vi "rest_get_latest.vi"(8 "error in (no error)":errorcluster, 11 "Base URL":string="http://localhost:5001/") -> (0 "error out":errorcluster, 2 "value":T1)   [LabVIEW 2024]
uses:
  <vilib>/addons/_JKI.lib/REST Client/classes/REST Client/REST Client.lvclass
  TypeDefs/MeasurementData.ctl
panel:
  out "Response body":string
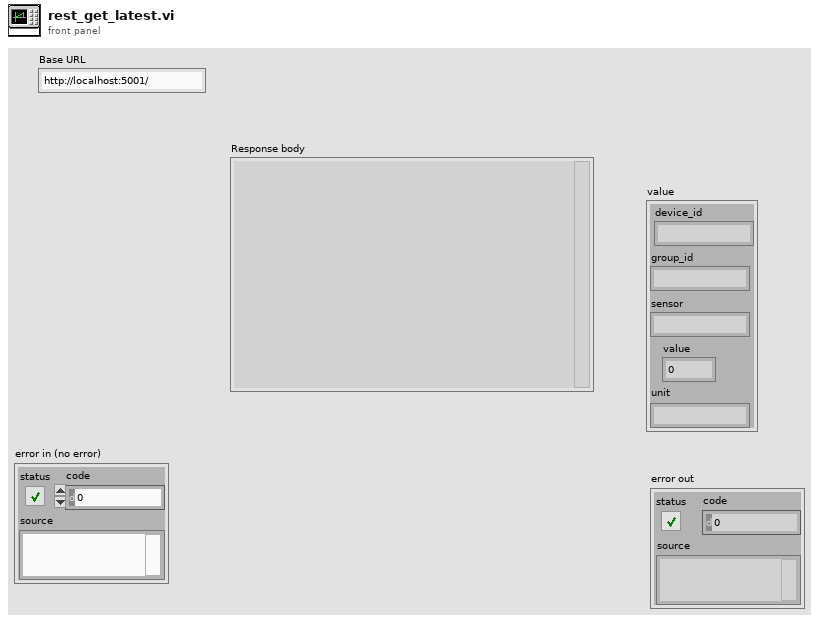
[diagram p1: front panel]
types:
  T1 = typedef "MeasurementData.ctl" = cluster{"device_id":string, "sensor":string, "value":dbl, "unit":string, "group_id":string}
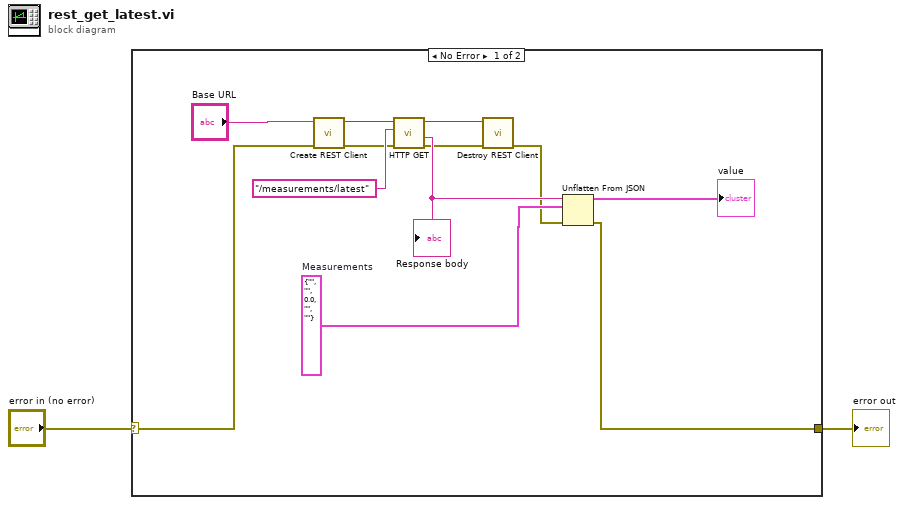
[diagram p0: block diagram]
diagram:
  n1 = case shown="No Error" "error in (no error)" {
    selector: "error in (no error)" -> [w7 w15]
    tunnel: [w3 w15] -> w1
    frame No Error {
      w9 = T1 {"device_id"="", "sensor"="", "value"=0.0, "unit"="", "group_id"=""}  # Measurements
      n2 = call <vilib>:"Create REST Client.vi"("error in (no error)"=w7, "Base URL"="Base URL") -> ("error out"=w6:errorcluster, "REST Client out"=w14:refnum<class "REST Client.lvclass">)  [unwired: 8 in]
      n3 = call-dynamic "HTTP GET.vi"("error in (no error)"=w6, "Path"="/measurements/latest", "REST Client in"=w14) -> ("error out"=w5:errorcluster, "Response body"=w10:string, "REST Client out"=w13:refnum<class "REST Client.lvclass">)  [unwired: 3 in, 3 out]
      "Response body" <- w10
      n4 = call-dynamic "Destroy REST Client.vi"("error in (no error)"=w5, "REST Client in"=w13) -> ("error out"=w4:errorcluster)  [unwired: 9 in]
      n5 = Unflatten From JSON(JSON string=w10, type and defaults=w9, error in (no error)=w4) -> (value=→"value":T1, error out=w3:errorcluster)  [unwired: 4 in]
    }
    frame Error {
    }
  }
  "error out" <- w1
